vi "Auto Warmup Shooter.vi"() -> ()   [LabVIEW 2015]
uses:
  Common Code/Shooter Commands.ctl
  Common Code/Shoot Modes Enum.ctl
  Common Code/Shot Type.ctl
  Robot Global Data.vi
panel:
  in  "Shot Type":i32
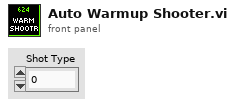
[diagram p1: front panel]
types:
  T1 = typedef "Shoot Modes Enum.ctl" = enum16{"Manual", "Safe", "Auto"}
  T2 = typedef "Shooter Commands.ctl" = enum16{"Idle", "Prime Shooter", "Shoot"}
  T3 = typedef "Shot Type.ctl" = enum16{"Batter Shot", "Corner Shot", "Curve Shot", "Vision Shot", "Deep Middle Shot"}
  T4 = typedef "Shooter Command Cluster.ctl" = cluster{"Command":T2, "Mode":T1, "Shot Type":T3, "Override Trigger Sensor":bool, "Override Angle?":bool}
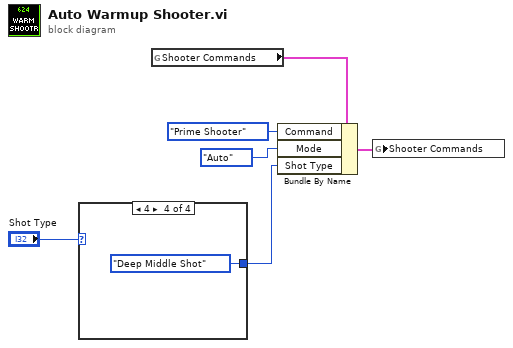
[diagram p0: block diagram]
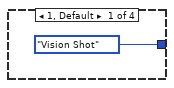
[diagram p2: hidden frame]
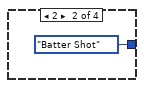
[diagram p3: hidden frame]
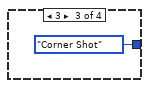
[diagram p4: hidden frame]
diagram:
  n1 = case shown="4" "Shot Type" {
    tunnel: [Shot_Type."Vision Shot" ("Shot Type") Shot_Type."Batter Shot" ("Shot Type") Shot_Type."Corner Shot" ("Shot Type") Shot_Type."Deep Middle Shot" ("Shot Type")] -> w3
    frame 1, Default {
    }
    frame 2 {
    }
    frame 3 {
    }
    frame 4 {
    }
  }
  n2 = global read "Robot Global Data.vi" "Shooter Commands"() -> (w4:T4)
  n3 = Bundle By Name(cluster=w4, "Command"=Shooter_Commands."Prime Shooter", "Mode"=Shoot_Modes_Enum."Auto", "Shot Type"=w3) -> (w5:T4)
  n4 = global write "Robot Global Data.vi" "Shooter Commands"(w5) -> ()
